vi "Create.vi"(8 "error in (no error)":errorcluster, 11 "ICPCON ET-7018i in":refnum<class "ICPCON ET-7018i.lvclass">) -> (0 "error out":errorcluster, 3 "ICPCON ET-7018i out":refnum<class "ICPCON ET-7018i.lvclass">)   [LabVIEW 2021, in "ICPCON ET-7018i.lvclass"]
uses:
  ICPCON ET-7018i.lvclass
  D:/my_projects/projects/Algorithms/Labview/21/Master CR/Master CR.lvclass
  Data Model/ICPCON ET7000 Data Model/ET-7018i/ET-7018i Data Model.lvclass
  D:/my_projects/projects/Algorithms/Labview/21/Modbus_v121c/Data Model/Device Data Model.lvclass
  Master CR.lvclass/Master CR.ctl
  TCP/TCP.lvclass
  ICPCON ET-7018i.lvclass/ICPCON ET-7018i.ctl
  Master CR.lvclass
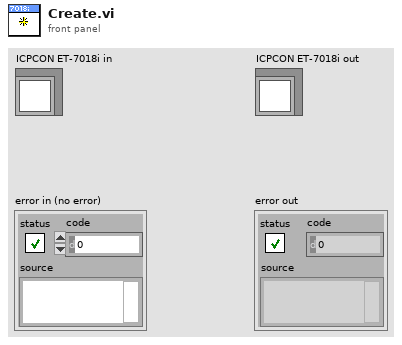
[diagram p1: front panel]
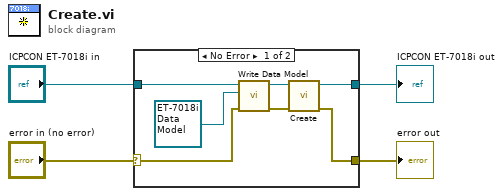
[diagram p0: block diagram]
diagram:
  n1 = case shown="No Error" "error in (no error)" {
    selector: "error in (no error)" -> [w5 w12]
    tunnel: [w9 w12] -> w3
    tunnel: [w10 w13] -> w4
    tunnel: "ICPCON ET-7018i in" -> [w11 w13]
    frame No Error {
      n2 = call "Write Data Model.vi"("error in (no error)"=w5, "Data Model"=refnum<class "ET-7018i Data Model.lvclass"> refnum ("Modbus API:Device Data Model"), "Master CR in"=w11) -> ("error out"=w8:errorcluster, "Master CR out"=w7:refnum<class "ICPCON ET-7018i.lvclass">)  [unwired: 7 in]
      n3 = call-parent "Create.vi"("error in (no error)"=w8, "TCP in"=w7) -> ("error out"=w9:errorcluster, "TCP out"=w10:refnum<class "ICPCON ET-7018i.lvclass">)  [unwired: 8 in]
    }
    frame Error {
    }
  }
  "error out" <- w3
  "ICPCON ET-7018i out" <- w4
